vi "ma_Estimate N and Alter BP.vi"(3 "type":T1(ring), 4 "nominal ripple":dbl=0.036315075773213946 format="%0.3e", 5 "sampling freq":dbl=1.0 format="%0.4f", 6 "Band Parameters In":T2(array[cluster])=[{"amplitude"=0.0, "lower freq"=0.0, "higher freq"=0.13333333333333333, "ripple weight"=1.0}, {"amplitude"=1.001, "lower freq"=0.16666666666666666, "higher freq"=0.3, "ripple weight"=1.0}, {"amplitude"=0.0, "lower freq"=0.3333333333333333, "higher freq"=0.5, "ripple weight"=1.0}] {"amplitude" format="%0.4f"; "lower freq" format="%0.4f"; "higher freq" format="%0.4f"; "ripple weight" format="%0.4f"}) -> (1 "Band Parameters Out":T2(array[cluster])=[{"amplitude"=0.0, "lower freq"=0.0, "higher freq"=0.13333333333333333, "ripple weight"=1.0}, {"amplitude"=1.001, "lower freq"=0.16666666666666666, "higher freq"=0.3, "ripple weight"=1.0}, {"amplitude"=0.0, "lower freq"=0.3333333333333333, "higher freq"=0.5, "ripple weight"=1.0}] {"amplitude" format="%0.4f"; "lower freq" format="%0.4f"; "higher freq" format="%0.4f"; "ripple weight" format="%0.4f"}, 2 "order":i32 min=0)   [LabVIEW 2020, in "NI_MAPro.lvlib"]
uses:
  NI_MAPro.lvlib
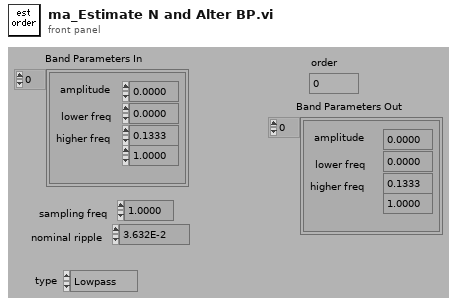
[diagram p1: front panel]
types:
  T1 = enum32{"Lowpass", "Highpass", "Bandpass", "Bandstop"}
  T2 = cluster{"amplitude":dbl, "lower freq":dbl, "higher freq":dbl, "ripple weight":dbl}[]
  T3 = cluster{"amplitude":dbl, "lower freq":dbl, "higher freq":dbl, "ripple weight":dbl}
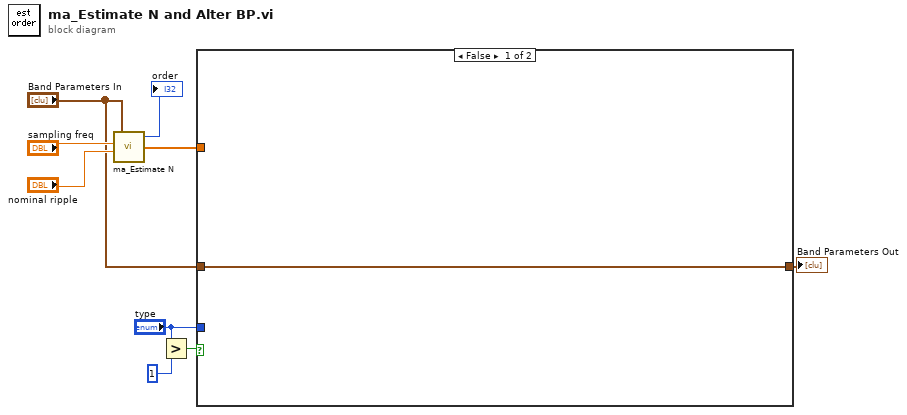
[diagram p0: block diagram]
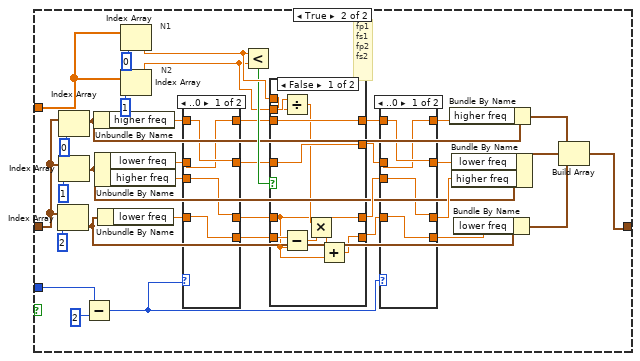
[diagram p2: hidden frame]
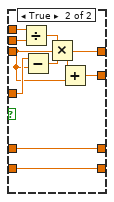
[diagram p4: hidden frame]
diagram:
  n1 = call "ma_Estimate N.vi"("nominal ripple"="nominal ripple", "sampling freq"="sampling freq", "Band Parameters In"="Band Parameters In") -> ("all orders"=w4:dbl[], "order"=→"order":i32)  [unwired: 2 in]
  n2 = Greater?(x="type", y=u32 1) -> (0:w1:bool)
  n3 = case shown="False" w1 {
    tunnel: "Band Parameters In" -> [w10 w43]
    tunnel: [w10 w11] -> w5
    tunnel: w4 -> [_ w34]
    tunnel: "type" -> [_ w42]
    frame False {
    }
    frame True {
      # "N2"
      # "N1"
      # "fp1\nfs1\nfp2\nfs2"
      n4 = Index Array(array=w43, index=2) -> (element=w15:T3)
      n5 = Index Array(array=w43, index=0) -> (element=w17:T3)
      n6 = Index Array(array=w43, index=1) -> (element=w16:T3)
      n7 = Subtract(x=w42, y=2) -> (x-y=w26:u32)
      n8 = Unbundle By Name(w17) -> ("higher freq"=w40:dbl)
      n9 = Unbundle By Name(w16) -> ("lower freq"=w39:dbl, "higher freq"=w37:dbl)
      n10 = Unbundle By Name(w15) -> ("lower freq"=w38:dbl)
      n11 = Index Array(array=w34, index=0) -> (element=w33:dbl)
      n12 = Index Array(array=w34, index=1) -> (element=w31:dbl)
      n13 = case shown="..0" w26 {
        tunnel: w40 -> [w78 w82]
        tunnel: [w77 w82] -> w30
        tunnel: w39 -> [w77 w81]
        tunnel: [w78 w81] -> w29
        tunnel: w38 -> [w75 w80]
        tunnel: [w76 w80] -> w28
        tunnel: [w75 w79] -> w27
        tunnel: w37 -> [w76 w79]
        frame ..0 {
        }
        frame 1.. {
        }
      }
      n14 = Less?(x=w33, y=w31) -> (x < y?=w32:bool)
      n15 = case shown="False" w32 {
        tunnel: w33 -> [w62 w74]
        tunnel: w31 -> [w63 w73]
        tunnel: w30 -> [w64 w65]
        tunnel: w29 -> [w61 w66]
        tunnel: w28 -> [w56 w68]
        tunnel: w27 -> [w58 w67]
        tunnel: [w64 w65] -> w25
        tunnel: [w61 w69] -> w24
        tunnel: [w56 w68] -> w23
        tunnel: [w55 w67] -> w22
        frame False {
          n16 = Divide(x=w63, y=w62) -> (x/y=w57:dbl)
          n17 = Subtract(x=w58, y=w56) -> (x-y=w60:dbl)
          n18 = Multiply(x=w57, y=w60) -> (x*y=w59:dbl)
          n19 = Add(x=w59, y=w56) -> (x+y=w55:dbl)
        }
        frame True {
          n20 = Divide(x=w74, y=w73) -> (x/y=w72:dbl)
          n21 = Subtract(x=w66, y=w65) -> (x-y=w71:dbl)
          n22 = Multiply(x=w72, y=w71) -> (x*y=w70:dbl)
          n23 = Add(x=w70, y=w65) -> (x+y=w69:dbl)
        }
      }
      n24 = case shown="..0" w26 {
        tunnel: w25 -> [w50 w54]
        tunnel: [w49 w54] -> w21
        tunnel: w24 -> [w49 w53]
        tunnel: [w50 w53] -> w20
        tunnel: w22 -> [w47 w52]
        tunnel: [w48 w52] -> w19
        tunnel: [w47 w51] -> w18
        tunnel: w23 -> [w48 w51]
        frame ..0 {
        }
        frame 1.. {
        }
      }
      n25 = Bundle By Name(cluster=w17, "higher freq"=w21) -> (w14:T3)
      n26 = Bundle By Name(cluster=w16, "lower freq"=w20, "higher freq"=w19) -> (w13:T3)
      n27 = Bundle By Name(cluster=w15, "lower freq"=w18) -> (w12:T3)
      n28 = Build Array(w14, w13, w12) -> (w11:T2)
    }
  }
  "Band Parameters Out" <- w5
